vi "Simultaneous_AI_AO.vi"() -> ()   [LabVIEW 2012]
doc: "I. Description:\nThis example demonstrates how to continuously acquire and generate data at the same time, synchronized with one another.\n\nII. Instructions for Running:\n1. Select the physical channel to correspond to where your signal is input on the DAQ device. Also, select the corresponding channel for where your signal is being generated.\n2. Enter the minimum and maximum voltage ranges.\nNote: For better accuracy try to match the input range to the expected voltage level of the measured signal.\n3. Set the sample rate of the acquisition.\nNote: The rate should be at least twice as fast as the maximum frequency component of the signal being acquired. \n6. Select the Rate for the generation\n7. Select what type of signal to generate and the amplitude.\nNote: This example requires two DMA channels to run. If your hardware does not support two DMA channels, you need to set the Data Transfer Mechanism property for the Analog Output Task to use \"Interrupts\". The Data Transfer Mechanism property is located in the DAQmx Channel Property hierarchy at:\n\nDAQmx Channel Property Node>>Analog Output>>General Properties>>Advanced>>Data Transfer and Memory>>Data Transfer Mechanism\n\nRefer to your device documentation to determine how many DMA channels are supported for your hardware.\n\nIII. Block Diagram Steps:\n1. Create an analog input voltage channel. Also, create an analog output voltage channel.\n2. Set the rate for the sample clock. Additionally, define the sample mode to be continuous. Also, set the sample clock rate for the signal generation.\n2a. Call the Get Terminal Name with Device Prefix VI. This will take a Task and a terminal and create a properly formatted device + terminal name to use as the source of the Trigger.\n3. Define the parameters for a Digital Edge Start Trigger. Set the Analog output to trigger off the AI Start Trigger. This is an internal trigger signal.\n4. Use the Basic Function Generator VI to create the signal to be generated.\n5. Call the Start VI to arm the two functions. Make sure the analog output is armed before the analog input. This will ensure both will start at the same time.\n6. Read the waveform data in a loop until the user hits the stop button or an error occurs. The Is Task Done? VI is used to check for errors in the Analog Output Task.\n7. Call the Clear VI to Clear the Task\n8. Use the popup dialog box to display an error if any.\n\nIV. I/O Connections Overview:\nMake sure your signal input/output terminals match the Physical Channel I/O controls."
uses:
  <vilib>/DAQmx/write.llb/DAQmx Write (Analog Wfm 1Chan NSamp).vi
  <vilib>/DAQmx/read.llb/DAQmx Read (Analog 1D Wfm NChan NSamp).vi
  <vilib>/DAQmx/create/channels.llb/DAQmx Create Channel (AI-Voltage-Basic).vi
  <vilib>/DAQmx/create/channels.llb/DAQmx Create Channel (AO-Voltage-Basic).vi
  <vilib>/DAQmx/configure/timing.llb/DAQmx Timing (Sample Clock).vi
  <vilib>/DAQmx/configure/trigger.llb/DAQmx Start Trigger (Digital Edge).vi
  <vilib>/Utility/file.llb/Write To Spreadsheet File (DBL).vi
  <vilib>/DAQmx/miscellaneous.llb/DAQmx Fill In Error Info.vi
  <vilib>/measure/NI_MABase.lvlib
  <resource>/objmgr/daqmx.rc
panel:
  in  "file path":path=path "c:/data.txt"
  in  "frequency":dbl=200.0 format="%0.2p"
  out "Time Domain":waveform(dbl)[](graph)
  in  "Sampling Info":T1={"Sampling Rate"=100000.0, "Number of Samples"=2400} {"Sampling Rate" format="%.2p"}
  in  "Amplitude":dbl=2.0 format="%0.2p"
  in  "Signal Type":T2(ring)=enum."Triangle Wave"
  in  "Channel":tag="Dev2/ao0" caption="Output Physical Channels"
  in  "Channel":tag="Dev2/ai1,Dev2/ai2" caption="Input Physical Channel"
  # "Channel Parameters"
  # "Signal Generation"
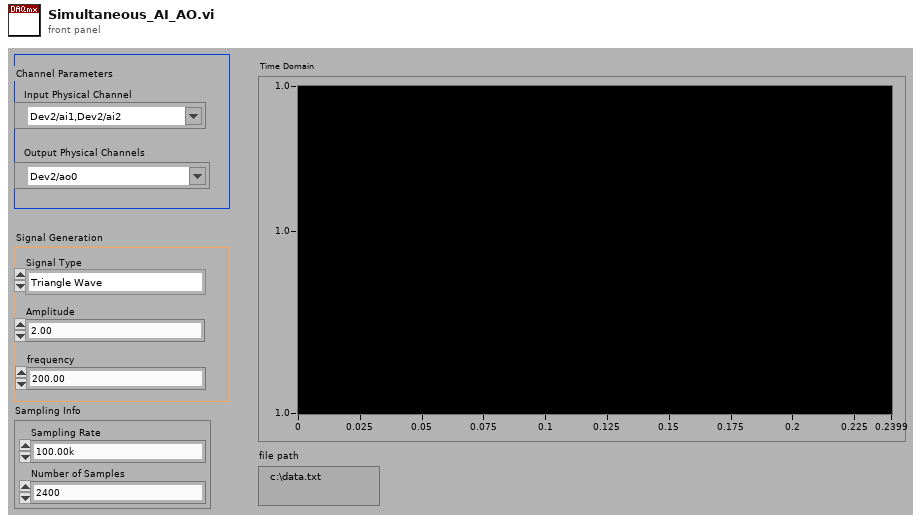
[diagram p1: front panel]
types:
  T1 = cluster{"Sampling Rate":dbl, "Number of Samples":u32}
  T2 = enum16{"Sine Wave", "Triangle Wave", "Square Wave", "Sawtooth Wave"}
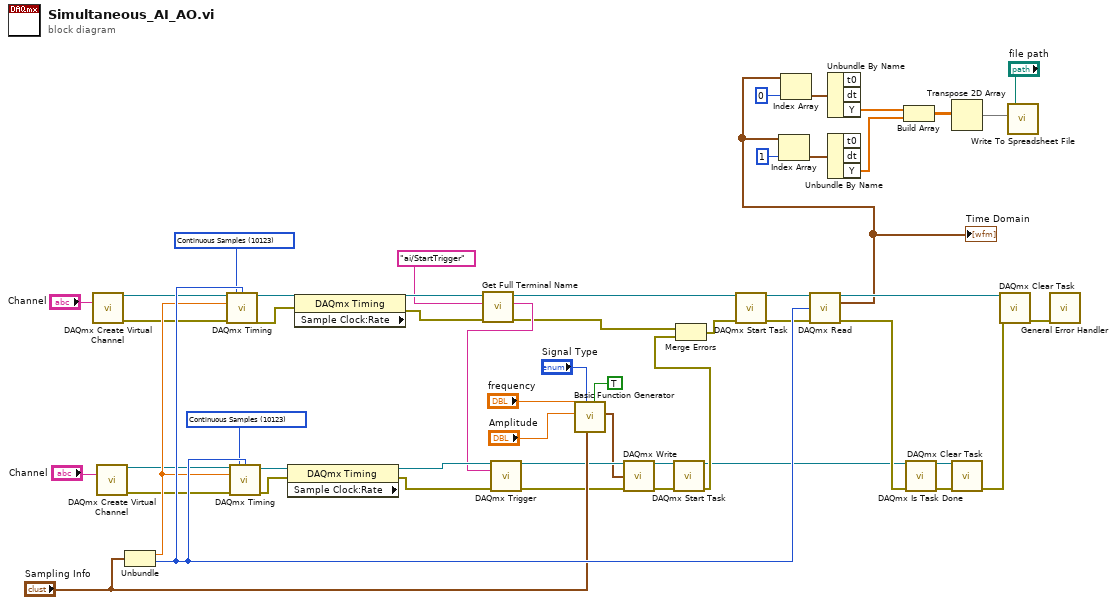
[diagram p0: block diagram]
diagram:
  w25 = 10123 items=["Finite Samples"=10178, "Continuous Samples"=10123] ("sample mode")
  w21 = 10123 items=["Finite Samples"=10178, "Continuous Samples"=10123] ("sample mode")
  n1 = call-poly <vilib>:"DAQmx Create Virtual Channel.vi"("physical channels"="Channel") -> ("task out"=w23:refnum<k21>, "error out"=w22:errorcluster)  [unwired: 13 in]
  n2 = call-poly <vilib>:"DAQmx Create Virtual Channel.vi"("physical channels"="Channel") -> ("task out"=w26:refnum<k21>, "error out"=w27:errorcluster)  [unwired: 13 in]
  n3 = Unbundle("Sampling Info") -> ("Sampling Rate"=w52:dbl, "Number of Samples"=w53:u32)
  n4 = call-poly <vilib>:"DAQmx Timing.vi"("task/channels in"=w23, "sample mode"=w21, "samples per channel"=w53, "rate"=w52, "error in"=w22) -> ("task out"=w45:refnum<k21>, "error out"=w46:errorcluster)  [unwired: 9 in]
  n5 = call-poly <vilib>:"DAQmx Timing.vi"("task/channels in"=w26, "sample mode"=w25, "samples per channel"=w53, "rate"=w52, "error in"=w27) -> ("task out"=w38:refnum<k21>, "error out"=w39:errorcluster)  [unwired: 9 in]
  n6 = property class="DAQmx Timing" props=["Sample Clock:Rate"](reference=w38, error in=w39) -> (reference out=w37:refnum<k21>, error out=w40:errorcluster)  [unwired: 1 out]
  n7 = property class="DAQmx Timing" props=["Sample Clock:Rate"](reference=w45, error in=w46) -> (reference out=w6:refnum<k21>, error out=w4:errorcluster)  [unwired: 1 out]
  n8 = call "Get Full Terminal Name.vi"("error in (no error)"=w4, "Local Terminal Name"="ai/StartTrigger" ("terminal"), "task/channels in"=w6) -> ("error out"=w1:errorcluster, "Terminal Name with Device Prefix"=w3:tag, "task out"=w2:refnum<k21>)  [unwired: 6 in]
  n9 = call-poly <vilib>:"DAQmx Trigger.vi"("task/channels in"=w37, "source"=w3, "error in"=w40) -> ("task out"=w33:refnum<k21>, "error out"=w32:errorcluster)  [unwired: 11 in]
  n10 = call <vilib>:"Basic Function Generator.vi"("reset signal"=TRUE, "sampling info"="Sampling Info", "signal type"="Signal Type", "amplitude"="Amplitude", "frequency"="frequency") -> ("signal out"=w18:waveform(dbl))  [unwired: 4 in, 2 out]
  n11 = call-poly <vilib>:"DAQmx Write.vi"("task/channels in"=w33, "data"=w18, "error in"=w32) -> ("task out"=w30:refnum<k21>, "error out"=w31:errorcluster)  [unwired: 10 in, 1 out]
  n12 = call <vilib>:"DAQmx Start Task.vi"("task/channels in"=w30, "error in"=w31) -> ("task out"=w28:refnum<k21>, "error out"=w42:errorcluster)  [unwired: 12 in]
  n13 = Merge Errors(w1, w42) -> (w43:errorcluster)
  n14 = call <vilib>:"DAQmx Start Task.vi"("task/channels in"=w2, "error in"=w43) -> ("task out"=w41:refnum<k21>, "error out"=w44:errorcluster)  [unwired: 12 in]
  n15 = call-poly <vilib>:"DAQmx Read.vi"("task/channels in"=w41, "number of samples per channel"=w53, "error in"=w44) -> ("task out"=w20:refnum<k21>, "data"=w7:waveform(dbl)[], "error out"=w50:errorcluster)  [unwired: 10 in]
  "Time Domain" <- w7
  n16 = Index Array(array=w7, index=1) -> (element=w11:waveform(dbl))
  n17 = Index Array(array=w7, index=0) -> (element=w13:waveform(dbl))
  n18 = Unbundle By Name(w13) -> ("Y"=w12:dbl[])  [unwired: 2 out]
  n19 = Unbundle By Name(w11) -> ("Y"=w10:dbl[])  [unwired: 2 out]
  n20 = Build Array(w12, w10) -> (w9:dbl[][])
  n21 = call <vilib>:"DAQmx Is Task Done.vi"("task/channels in"=w28, "error in"=w50) -> ("task out"=w29:refnum<k21>, "error out"=w47:errorcluster)  [unwired: 11 in, 1 out]
  n22 = Transpose 2D Array(2D array=w9) -> (transposed array=w8:dbl[][])
  n23 = call <vilib>:"DAQmx Clear Task.vi"("task in"=w29, "error in"=w47) -> ("error out"=w48:errorcluster)  [unwired: 13 in]
  n24 = call <vilib>:"DAQmx Clear Task.vi"("task in"=w20, "error in"=w48) -> ("error out"=w49:errorcluster)  [unwired: 13 in]
  n25 = call-poly <vilib>:"Write To Spreadsheet File.vi"("2D data"=w8, "file path (dialog if empty)"="file path") -> ()  [unwired: 6 in, 1 out]
  n26 = call <vilib>:"General Error Handler.vi"("error in (no error)"=w49) -> ()  [unwired: 10 in, 5 out]
